vi "Practica01.vi"() -> ()   [LabVIEW 2020]
panel:
  in  "stop":bool
  out "Waveform Chart 2":dbl(graph)
  out "Waveform Chart":dbl(graph)
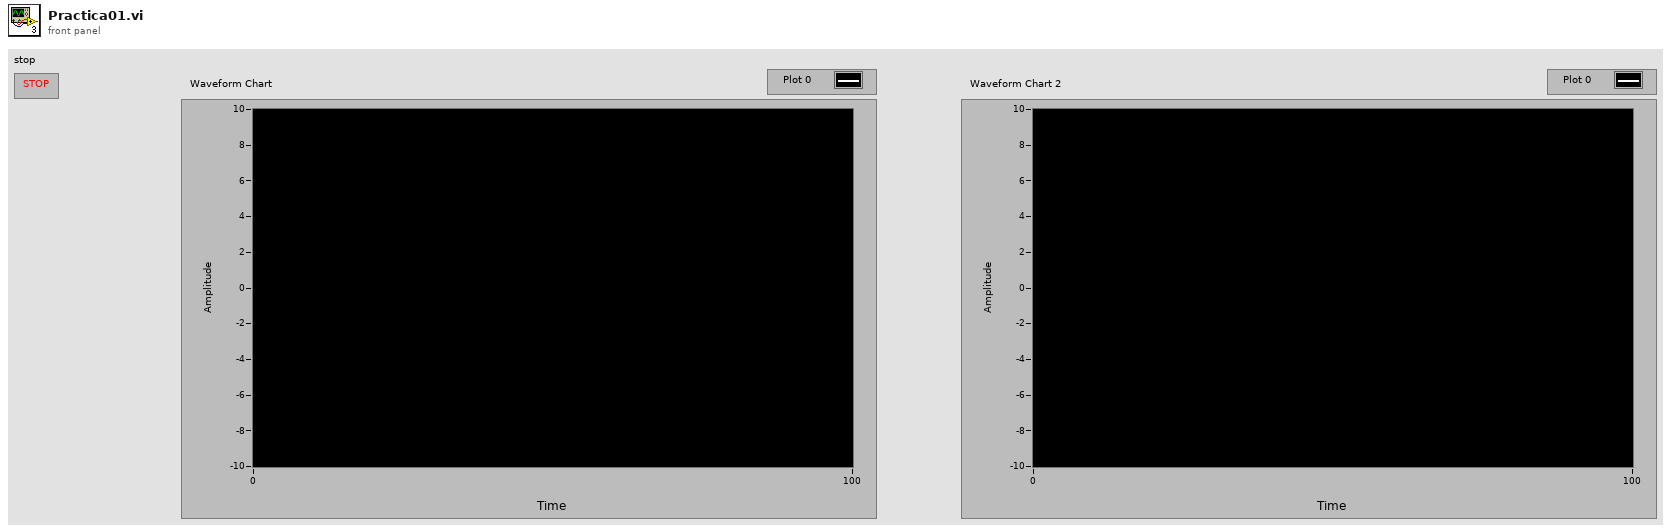
[diagram p1: front panel]
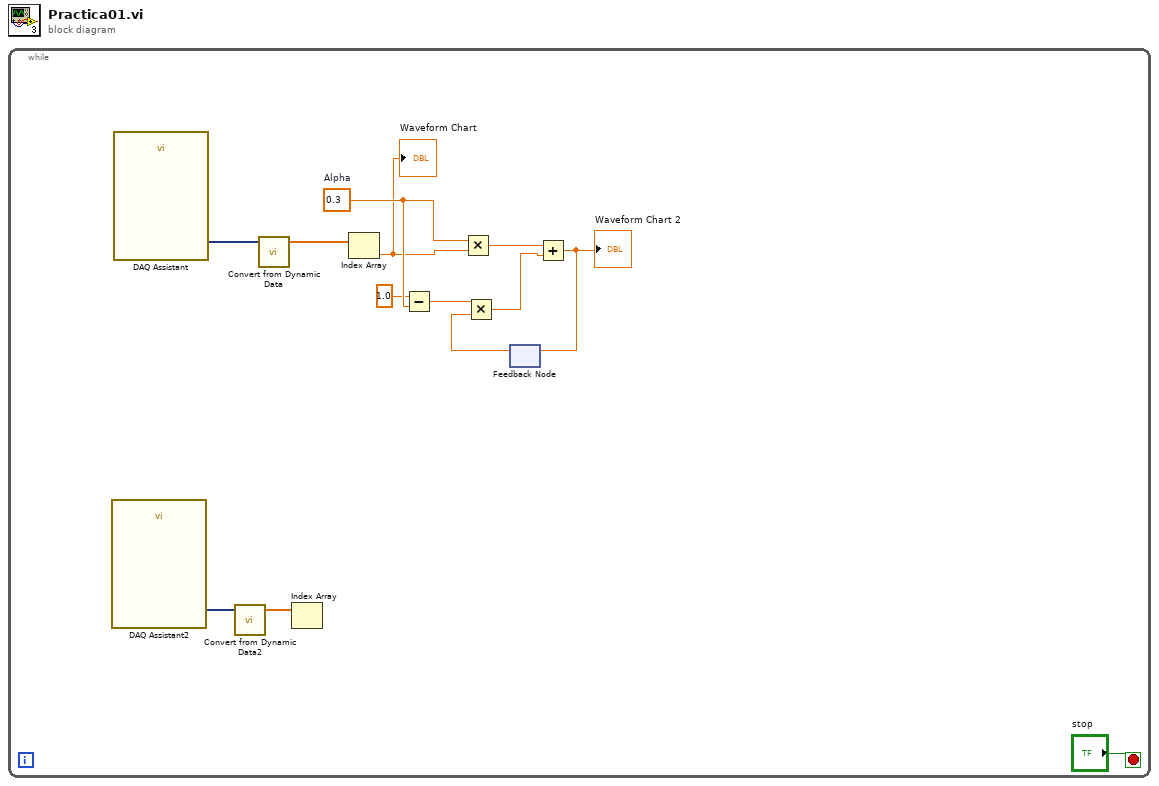
[diagram p0: block diagram]
diagram:
  n1 = while {
    stop <- "stop" stop-if-true
    w11 = 0.3  # Alpha
    n2 = call "DAQ Assistant2"() -> ("data"=w2:dynamicdata)  [unwired: 17 in, 2 out]
    n3 = call "DAQ Assistant"() -> ("data"=w7:dynamicdata)  [unwired: 17 in, 2 out]
    n4 = call "Convert from Dynamic Data2"("Dynamic Data Type"=w2) -> ("Array"=w1:dbl[])  [unwired: 3 in]
    n5 = call "Convert from Dynamic Data"("Dynamic Data Type"=w7) -> ("Array"=w6:dbl[])  [unwired: 3 in]
    n6 = Index Array "Index Array"(array=w1) -> ()  [unwired: 1 in, 1 out]
    n7 = Index Array "Index Array"(array=w6) -> (element=w5:dbl)  [unwired: 1 in]
    "Waveform Chart" <- w5
    n8 = Subtract(x=1.0, y=w11) -> (x-y=w12:dbl)
    n9 = Multiply(x=w11, y=w5) -> (x*y=w9:dbl)
    n10 = feedback #1() -> (w13:dbl)  [unwired: 1 in]
    n11 = Multiply(x=w12, y=w13) -> (x*y=w8:dbl)
    n12 = Add(x=w9, y=w8) -> (x+y=w4:dbl)
    "Waveform Chart 2" <- w4
    n13 = feedback-in #1(w4) -> ()
  }
